vi "update_altitud.vi"(7 "LabVIEW Web Service Request":refnum<class "Web Request.lvclass">) -> ()   [LabVIEW 2014]
uses:
  <vilib>/wsapi/Web Request.lvclass
  Globals/globalAntena.vi
panel:
  out "AntenaAltitud":dbl
  # "Use the Web Service Request input terminal to call the VIs on the Web Services palette. Do not remove it from the connector pane unless you don't need access to the palette."
  # "Each additional control wired to the connector pane will be available as an input in the URL. To include an indicator in terminal-mode output (the default setting), it must also be wired to the connector pane."
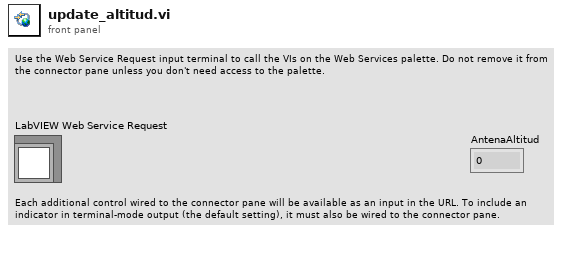
[diagram p1: front panel]
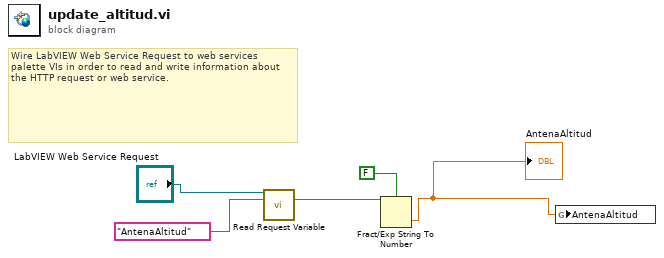
[diagram p0: block diagram]
diagram:
  # "Wire LabVIEW Web Service Request to web services palette VIs in order to read and write information about the HTTP request or web service."
  n1 = call <vilib>:"Read Request Variable.vi"("LabVIEW Web Service Request"="LabVIEW Web Service Request", "variable name"="AntenaAltitud") -> ("value"=w3:string)  [unwired: 11 in, 2 out]
  n2 = Fract/Exp String To Number(use system decimal point (T)=FALSE, string=w3) -> (number=w1:dbl)  [unwired: 2 in, 1 out]
  "AntenaAltitud" <- w1
  n3 = global write "globalAntena.vi" "AntenaAltitud"(w1) -> ()
